vi "Set Item.vi"(6 "$Path or Item Name":string, 7 "error in (no error)":errorcluster, 8 "JSON to Insert":string, 9 "Offset":i32, 10 "JSON":string="{}") -> (0 "error out":errorcluster, 1 "Replaced":bool, 3 "<JSON>":string)   [LabVIEW 2021, in "json.facade.lvlib"]
doc: "Insert or replace JSON item at the $Path specified. Only sets the first found item at the $Path."
uses:
  json.facade.lvlib
  jsontext/JSONtext.lvlib
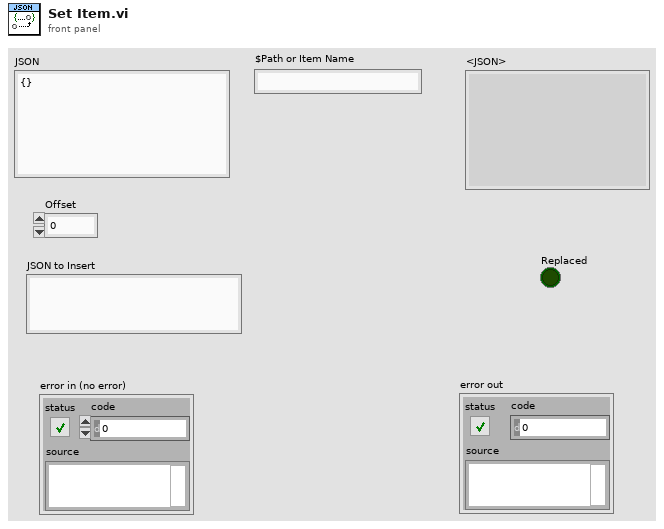
[diagram p1: front panel]
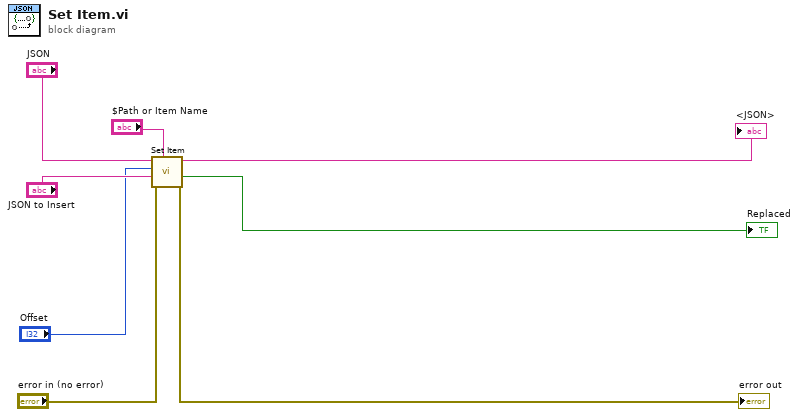
[diagram p0: block diagram]
diagram:
  n1 = call "Set Item.vi"("$Path or Item Name"="$Path or Item Name", "error in (no error)"="error in (no error)", "JSON to Insert"="JSON to Insert", "Offset"="Offset", "JSON"="JSON") -> ("error out"=→"error out":errorcluster, "Replaced"=→"Replaced":bool, "<JSON>"=→"<JSON>":string)  [unwired: 3 in]
